vi "get_temp.vi"(10 "错误输入（无错误）":errorcluster, 11 "VISA资源名称":refnum<visa-resource-name>="COM4") -> (1 "error out":errorcluster caption="错误输出", 2 "实时温度":dbl, 3 "VISA资源名称输出":refnum<visa-resource-name>)   [LabVIEW 2017]
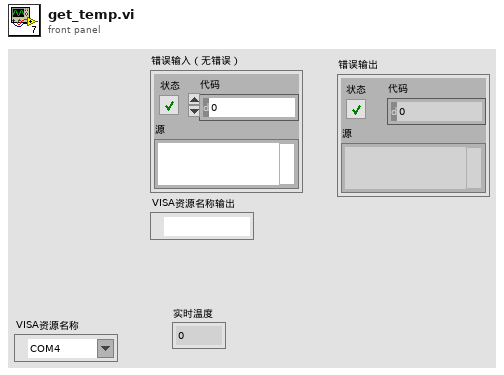
[diagram p1: front panel]
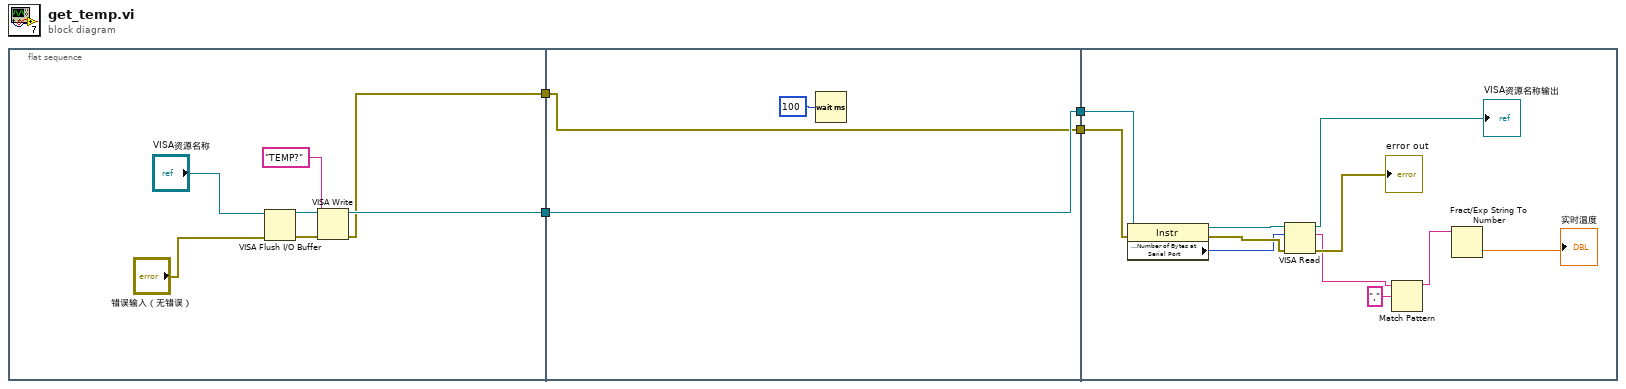
[diagram p0: block diagram]
diagram:
  n1 = flat-sequence {
    tunnel: [w8] -> w4
    tunnel: [w7] -> w3
    tunnel: w4 -> [w13]
    tunnel: w3 -> [w12]
    tunnel: [w13] -> w2
    tunnel: [w12] -> w1
    tunnel: w2 -> [w21]
    tunnel: w1 -> [w20]
    frame #0 {
      n2 = VISA Flush I/O Buffer(VISA resource name="VISA资源名称", error in (no error)="错误输入（无错误）") -> (VISA resource name out=w10:refnum<visa-resource-name>, error out=w11:errorcluster)  [unwired: 1 in]
      n3 = VISA Write(VISA resource name=w10, write buffer="TEMP?" ("写入缓冲区"), error in (no error)=w11) -> (VISA resource name out=w8:refnum<visa-resource-name>, error out=w7:errorcluster)  [unwired: 1 out]
    }
    frame #1 {
      n4 = Wait (ms)(milliseconds to wait=u32 100 ("等待时间（毫秒）")) -> ()  [unwired: 1 out]
    }
    frame #2 {
      n5 = property class="Instr"(reference=w21, error in=w20) -> (reference out=w25:refnum<visa-resource-name>, error out=w24:errorcluster, "Serial Settings:Number of Bytes at Serial Port"=w23:u32)
      n6 = VISA Read(VISA resource name=w25, byte count=w23, error in (no error)=w24) -> (VISA resource name out=→"VISA资源名称输出":refnum<visa-resource-name>, read buffer=w16:string, error out=→"error out":errorcluster)  [unwired: 1 out]
      n7 = Match Pattern(string=w16, regular expression="," ("正则表达式")) -> (before substring=w15:string)  [unwired: 1 in, 3 out]
      n8 = Fract/Exp String To Number(string=w15) -> (number=→"实时温度":dbl)  [unwired: 3 in, 1 out]
    }
  }
